vi "Get Joystick 2015.vi"() -> (3 "Robot Controls":T1)   [LabVIEW 2014]
uses:
  Subsystem VIs/Robot Control Outputs.ctl
  Global Variables/Refnum Names.vi
  <vilib>/Rock Robotics/WPI/Joystick/WPI_JoystickGetSetRefNum.vi
  <vilib>/Rock Robotics/Network Tables/SD Write Numeric Array.vi
  <vilib>/Rock Robotics/Network Tables/SD Write Boolean Array.vi
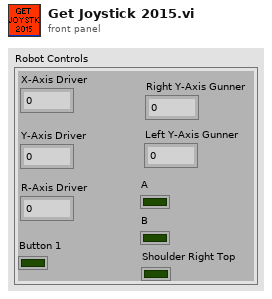
[diagram p1: front panel]
types:
  T1 = typedef "Robot Control Outputs.ctl" = cluster{"X-Axis Driver":dbl, "Y-Axis Driver":dbl, "R-Axis Driver":dbl, "Button 1":bool, "Right Y-Axis Gunner":dbl, "Left Y-Axis Gunner":dbl, "A":bool, "B":bool, "Shoulder Right Top ":bool}
  T2 = typedef "WPI_JoystickDevRef.ctl" = cluster{"Device":T3}
  T3 = typedef "WPI_JoystickDeviceEnum.ctl" = enum16{"USB 0", "USB 1", "USB 2", "USB 3", "USB 4", "USB 5"}
  T4 = cluster{"Axes[0]":dbl, "Axes[1]":dbl, "Axes[2]":dbl, "Axes[3]":dbl, "Axes[4]":dbl, "Axes[5]":dbl, "Axes[6]":dbl, "Axes[7]":dbl, "Axes[8]":dbl}
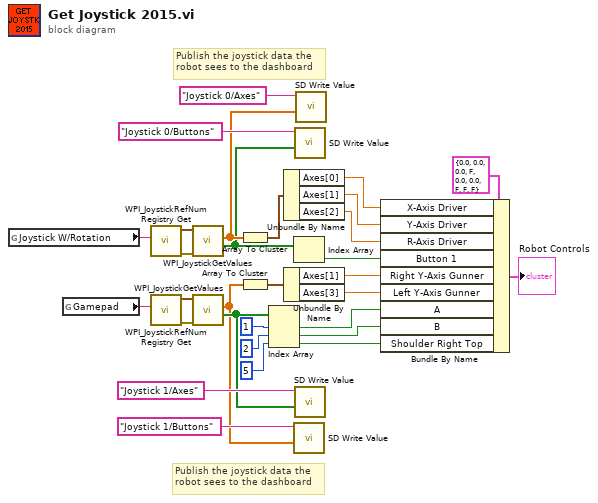
[diagram p0: block diagram]
diagram:
  # "Publish the joystick data the\nrobot sees to the dashboard"
  # "Publish the joystick data the\nrobot sees to the dashboard"
  n1 = global read "Refnum Names.vi" "Joystick W/Rotation"() -> (w28:string)
  n2 = global read "Refnum Names.vi" "Gamepad"() -> (w27:string)
  n3 = call <vilib>:"WPI_JoystickRefNum Registry Get.vi"("refnum name"=w28) -> ("error out"=w30:errorcluster, "JoystickDevRef"=w29:T2)  [unwired: 9 in]
  n4 = call <vilib>:"WPI_JoystickRefNum Registry Get.vi"("refnum name"=w27) -> ("error out"=w25:errorcluster, "JoystickDevRef"=w26:T2)  [unwired: 9 in]
  n5 = call <vilib>:"WPI_JoystickGetValues.vi"("error in (no error)"=w30, "JoystickDevRef"=w29) -> ("Buttons"=w6:bool[], "Axes"=w7:dbl[])  [unwired: 5 in, 3 out]
  n6 = call <vilib>:"WPI_JoystickGetValues.vi"("error in (no error)"=w25, "JoystickDevRef"=w26) -> ("Buttons"=w2:bool[], "Axes"=w1:dbl[])  [unwired: 5 in, 3 out]
  n7 = Array To Cluster(array=w7) -> (cluster=w24:T4)
  n8 = Array To Cluster(array=w1) -> (cluster=w23:T4)
  n9 = Index Array(array=w2, index #1=1 ("index"), index #2=2 ("index"), index #3=5 ("index")) -> (element #1=w13:bool, element #2=w12:bool, element #3=w11:bool)
  n10 = Unbundle By Name(w24) -> ("Axes[0]"=w22:dbl, "Axes[1]"=w21:dbl, "Axes[2]"=w20:dbl)
  n11 = Unbundle By Name(w23) -> ("Axes[1]"=w18:dbl, "Axes[3]"=w17:dbl)
  n12 = Index Array(array=w6) -> (element=w19:bool)  [unwired: 1 in]
  n13 = call-poly <vilib>:"SD Write Value.vi"("Numeric Array"=w1, "Name"="Joystick 1/Buttons") -> ()  [unwired: 8 in, 2 out]
  n14 = call-poly <vilib>:"SD Write Value.vi"("Boolean Array"=w6, "Name"="Joystick 0/Buttons") -> ()  [unwired: 8 in, 2 out]
  n15 = call-poly <vilib>:"SD Write Value.vi"("Boolean Array"=w2, "Name"="Joystick 1/Axes") -> ()  [unwired: 8 in, 2 out]
  n16 = call-poly <vilib>:"SD Write Value.vi"("Numeric Array"=w7, "Name"="Joystick 0/Axes") -> ()  [unwired: 8 in, 2 out]
  n17 = Bundle By Name(cluster=T1 {"X-Axis Driver"=0.0, "Y-Axis Driver"=0.0, "R-Axis Driver"=0.0, "Button 1"=FALSE, "Right Y-Axis Gunner"=0.0, "Left Y-Axis Gunner"=0.0, "A"=FALSE, "B"=FALSE, "Shoulder Right Top "=FALSE} ("Driver/Gunner Controls"), "X-Axis Driver"=w22, "Y-Axis Driver"=w21, "R-Axis Driver"=w20, "Button 1"=w19, "Right Y-Axis Gunner"=w18, "Left Y-Axis Gunner"=w17, "A"=w13, "B"=w12, "Shoulder Right Top"=w11) -> (→"Robot Controls":T1)
